vi "decodeStream.vi"(8 "error in (no error)":errorcluster, 9 "beginIndex":i32, 10 "binary stream":u8[](array[numeric]), 11 "tBSONElement in":refnum<class "tBSONElement.lvclass">) -> (0 "error out":errorcluster, 1 "endIndex":i32, 2 "binary stream out":u8[](array[numeric]), 3 "tBSONElement out":refnum<class "tBSONElement.lvclass">)   [LabVIEW 2013, in "BSON.lvlib" / "tBSONElement.lvclass"]
doc: "Decodes a BSON element from a byte stream at a given offset."
uses:
  tBSONElement.lvclass
  status.ctl
  setName.vi
  BSON.lvlib
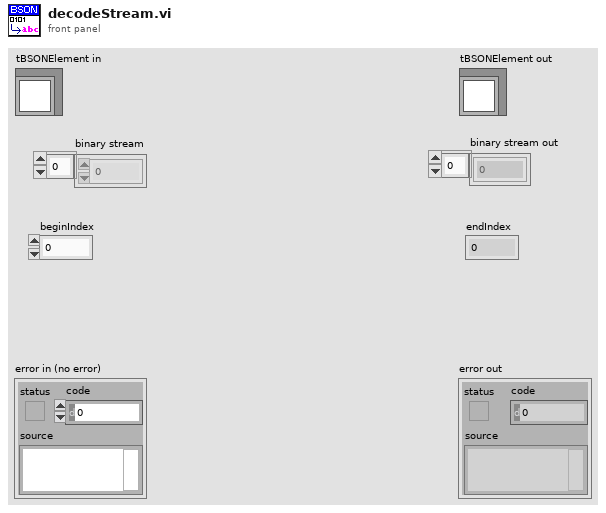
[diagram p1: front panel]
types:
  T1 = typedef "BSON.lvlib/status.ctl" = enum16{"Stream Corrupted or Ended Abruptly", "Incorrect Type In Stream", "ObjectID Invalid", "Method Not Implemented", "Invalid Name", "Invalid URI", "AutoReconnect", "Operation Failed", "Incorrectly Configured", "Cursor Not Found", "Timeout", "Invalid Type", "Empty Name", "Duplicate Name", "MD5Incorrect"}
  T2 = typedef "BSON.lvlib/tBSONElement.lvclass/type.ctl" = u8
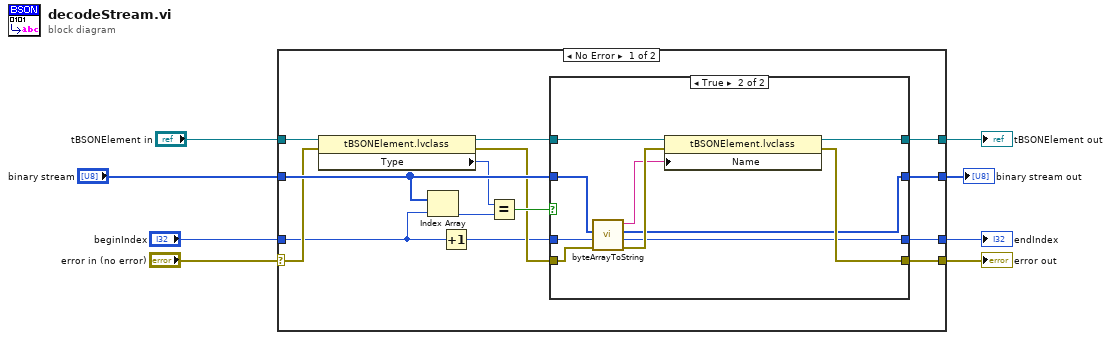
[diagram p0: block diagram]
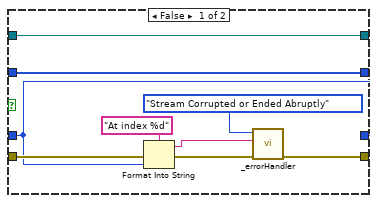
[diagram p2: hidden frame]
diagram:
  n1 = case shown="No Error" "error in (no error)" {
    selector: "error in (no error)" -> [w15 w45]
    tunnel: [w22 w45] -> w7
    tunnel: [w20 w44] -> w5
    tunnel: "tBSONElement in" -> [w17 w44]
    tunnel: "binary stream" -> [w19 w42]
    tunnel: "beginIndex" -> [w11 w43]
    tunnel: [w21 w43] -> w2
    tunnel: [w9 w42] -> w1
    frame No Error {
      n2 = property class="tBSONElement.lvclass"(reference=w17, error in=w15) -> (reference out=w16:refnum<class "tBSONElement.lvclass">, error out=w12:errorcluster, "Type"=w14:T2)
      n3 = Index Array(array=w19, index=w11) -> (element=w18:u8)
      n4 = Increment(x=w11) -> (x+1=w10:i32)
      n5 = Equal?(x=w14, y=w18) -> (x = y?=w13:bool)
      n6 = case shown="True" w13 {
        tunnel: [w30 w41] -> w22
        tunnel: [w24 w35] -> w21
        tunnel: [w29 w40] -> w20
        tunnel: w19 -> [w23 w38]
        tunnel: w16 -> [w29 w39]
        tunnel: w10 -> [w24 w34]
        tunnel: w12 -> [w28 w37]
        tunnel: [w23 w32] -> w9
        frame False {
          n7 = Format Into String(format string="At index %d", error in=w28, w24) -> (resulting string=w25:string, error out=w26:errorcluster)  [unwired: 1 in]
          n8 = call "_errorHandler.vi"("error in (no error)"=w26, "Additional Text"=w25, "Error Type"=status."Stream Corrupted or Ended Abruptly") -> ("error out"=w30:errorcluster)  [unwired: 8 in]
        }
        frame True {
          n9 = call "byteArrayToString.vi"("error in (no error)"=w37, "startIndex"=w34, "ByteArrayIn"=w38) -> ("error out"=w36:errorcluster, "endIndex"=w35:i32, "ByteArrayOut"=w32:u8[], "String"=w33:string)  [unwired: 5 in]
          n10 = property class="tBSONElement.lvclass"(reference=w39, error in=w36, "Name"=w33) -> (reference out=w40:refnum<class "tBSONElement.lvclass">, error out=w41:errorcluster)
        }
      }
    }
    frame Error {
    }
  }
  "error out" <- w7
  "tBSONElement out" <- w5
  "binary stream out" <- w1
  "endIndex" <- w2
